vi "Temp Conversion.vi"() -> ()   [LabVIEW 2014]
panel:
  in  "C-F Temp":dbl
  in  "C-K Temp":dbl
  in  "F-K Temp":dbl
  out "C-F Fahrenheit":dbl
  out "C-K Kelvin":dbl
  out "F-K Kelvin":dbl
  out "F-C Celsius":dbl
  in  "F-C Temp":dbl
  in  "If F-C Put 0\nIf F-K Put 1\nIf C-K Put 2\nIf C-F Put 3":dbl
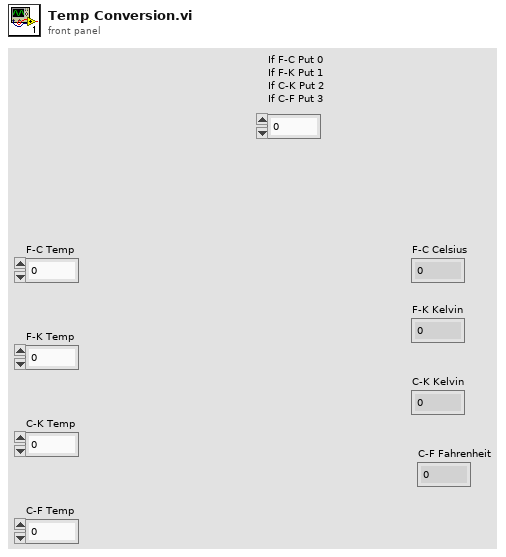
[diagram p1: front panel]
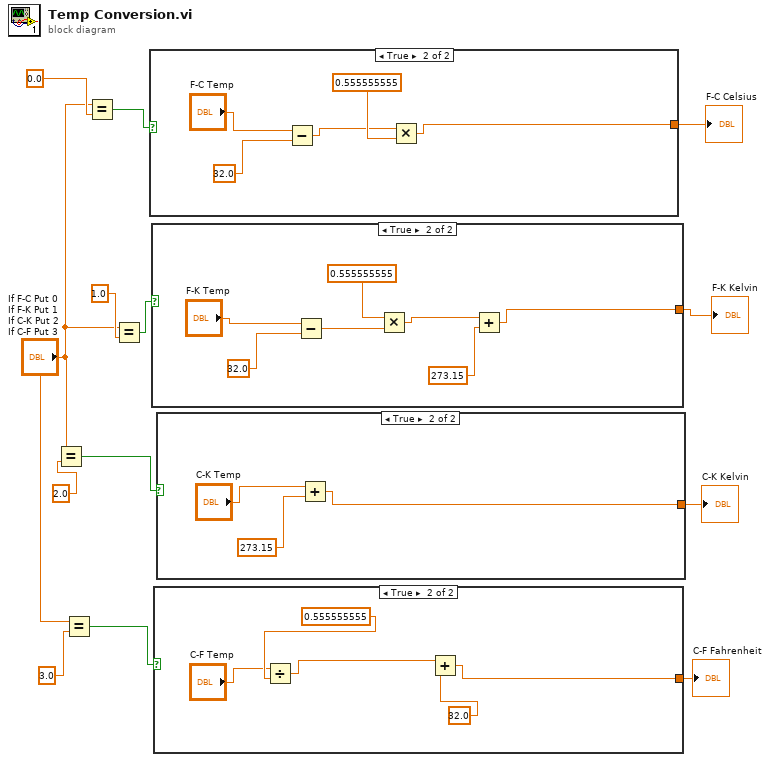
[diagram p0: block diagram]
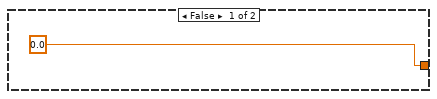
[diagram p2: hidden frame]
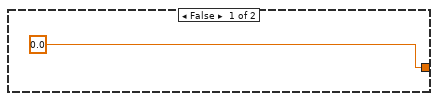
[diagram p3: hidden frame]
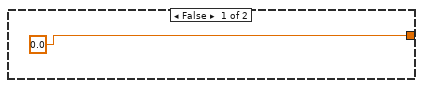
[diagram p4: hidden frame]
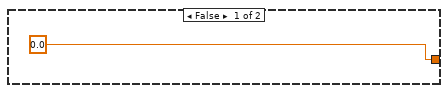
[diagram p5: hidden frame]
diagram:
  n1 = Equal?(x="If F-C Put 0\nIf F-K Put 1\nIf C-K Put 2\nIf C-F Put 3", y=2.0) -> (x = y?=w6:bool)
  n2 = Equal?(x="If F-C Put 0\nIf F-K Put 1\nIf C-K Put 2\nIf C-F Put 3", y=3.0) -> (x = y?=w5:bool)
  n3 = Equal?(x="If F-C Put 0\nIf F-K Put 1\nIf C-K Put 2\nIf C-F Put 3", y=0.0) -> (x = y?=w7:bool)
  n4 = Equal?(x="If F-C Put 0\nIf F-K Put 1\nIf C-K Put 2\nIf C-F Put 3", y=1.0) -> (x = y?=w8:bool)
  n5 = case shown="True" w7 {
    tunnel: [0.0 w15] -> w4
    frame False {
    }
    frame True {
      n6 = Subtract(x="F-C Temp", y=32.0) -> (x-y=w16:dbl)
      n7 = Multiply(x=w16, y=0.555555555) -> (x*y=w15:dbl)
    }
  }
  "F-C Celsius" <- w4
  n8 = case shown="True" w8 {
    tunnel: [0.0 w21] -> w3
    frame False {
    }
    frame True {
      n9 = Subtract(x="F-K Temp", y=32.0) -> (x-y=w25:dbl)
      n10 = Multiply(x=0.555555555, y=w25) -> (x*y=w22:dbl)
      n11 = Add(x=w22, y=273.15) -> (x+y=w21:dbl)
    }
  }
  "F-K Kelvin" <- w3
  n12 = case shown="True" w5 {
    tunnel: [0.0 w29] -> w1
    frame False {
    }
    frame True {
      n13 = Divide(x="C-F Temp", y=0.555555555) -> (x/y=w30:dbl)
      n14 = Add(x=w30, y=32.0) -> (x+y=w29:dbl)
    }
  }
  "C-F Fahrenheit" <- w1
  n15 = case shown="True" w6 {
    tunnel: [0.0 w35] -> w2
    frame False {
    }
    frame True {
      n16 = Add(x="C-K Temp", y=273.15) -> (x+y=w35:dbl)
    }
  }
  "C-K Kelvin" <- w2
